vi "Facade.vi"(0 "Data In":T5, 2 "Display State In":T3, 3 "Container State":T4) -> (6 "Data Out":T5, 7 "Display State Out":T3, 8 "Action":T2)   [LabVIEW 2020, in "Advanced Stimulus Options.xctl"]
uses:
  Advanced Stimulus Options.xctl
  Advanced Stimulus Options.ctl
  <vilib>/_xctls/Container State.ctl
  State.ctl
  <vilib>/_xctls/Action.ctl
  Utility VIs/Buttons/KCheckmarkBoolean 2.ctl
  <vilib>/_xctls/XControlSupport.lvlib
panel:
  in  "Persist":T1
  in  "Alternate polarity":T1
  in  "Expression":string
  in  "Variable":u16(ring)
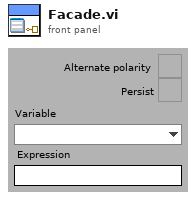
[diagram p1: front panel]
types:
  T1 = typedef "KCheckmarkBoolean 2.ctl" = bool
  T2 = typedef "XControlSupport.lvlib/Action.ctl" = cluster{"Data Changed?":bool, "State Changed?":bool, "Action Name":string}
  T3 = typedef "Advanced Stimulus Options.xctl/State.ctl" = cluster{"VarNames":string[], "show vars":bool, "show persist":bool}
  T4 = typedef "XControlSupport.lvlib/Container State.ctl" = cluster{"Indicator?":bool, "Run Mode?":bool, " Refnum":refnum<vi>}
  T5 = typedef "Advanced Stimulus Options.xctl/Advanced Stimulus Options.ctl" = cluster{"Rep Mask":string, "AltPol":bool, "Var":string, "Expr":string, "Persist":bool}
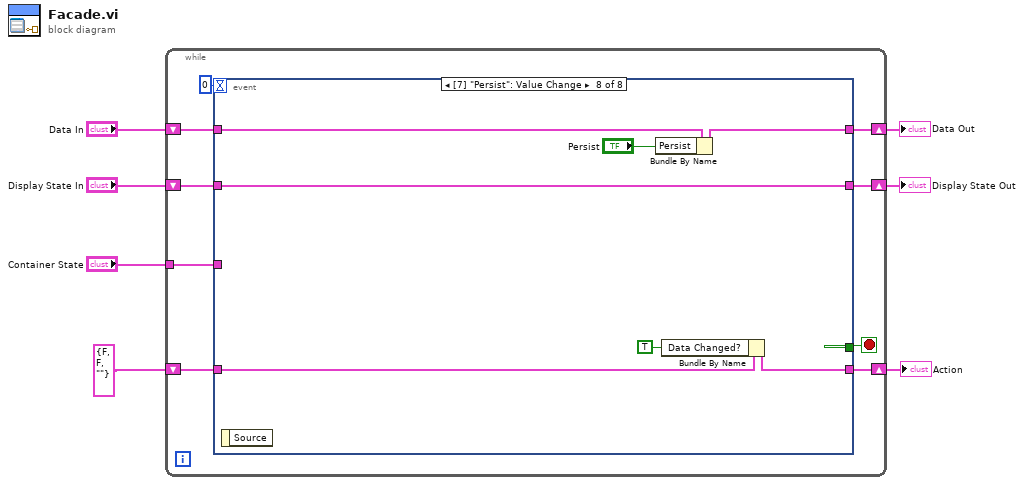
[diagram p0: block diagram]
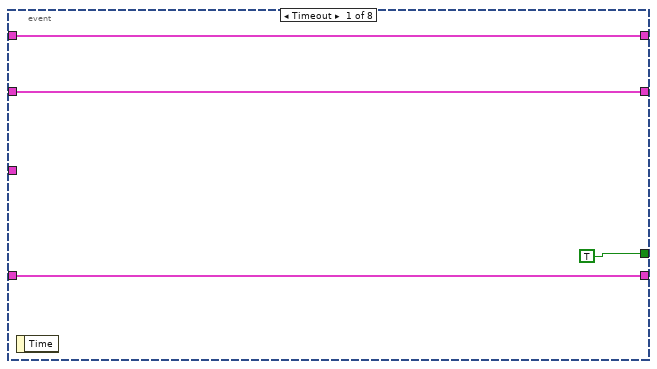
[diagram p2: hidden frame]
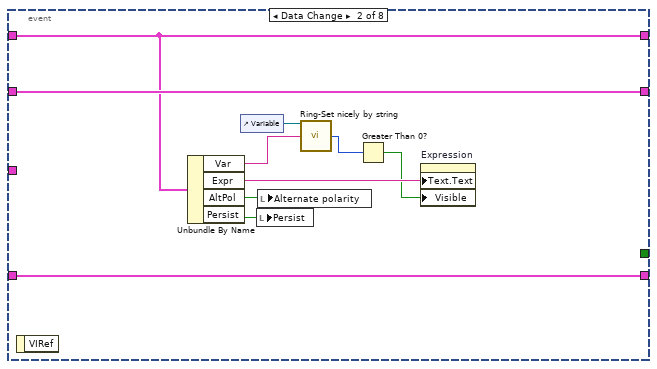
[diagram p3: hidden frame]
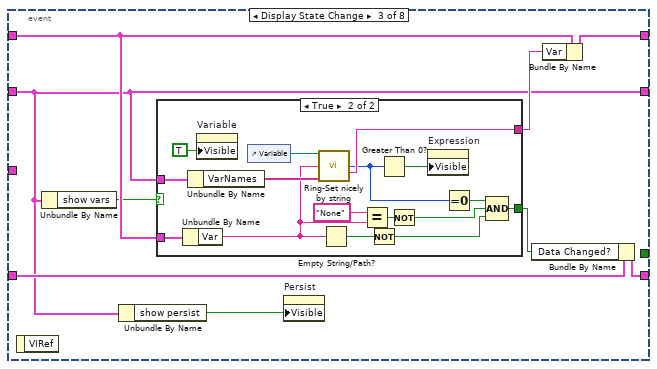
[diagram p4: hidden frame]
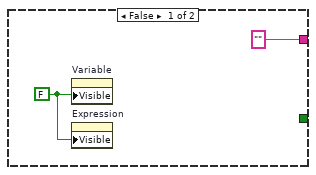
[diagram p5: hidden frame]
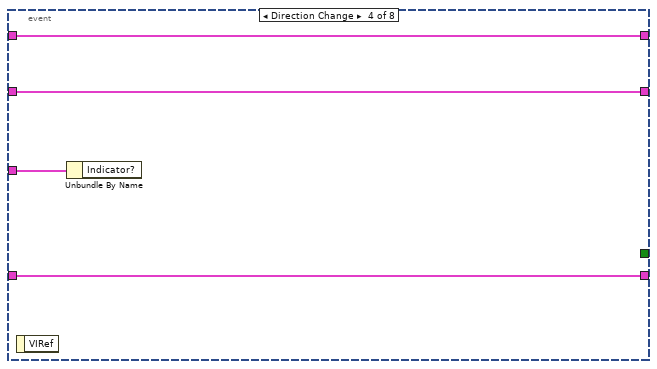
[diagram p6: hidden frame]
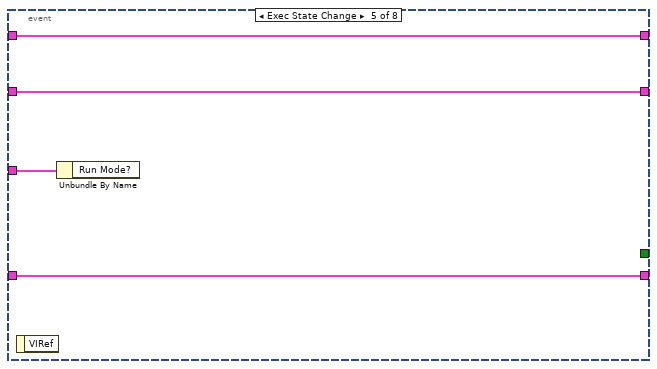
[diagram p7: hidden frame]
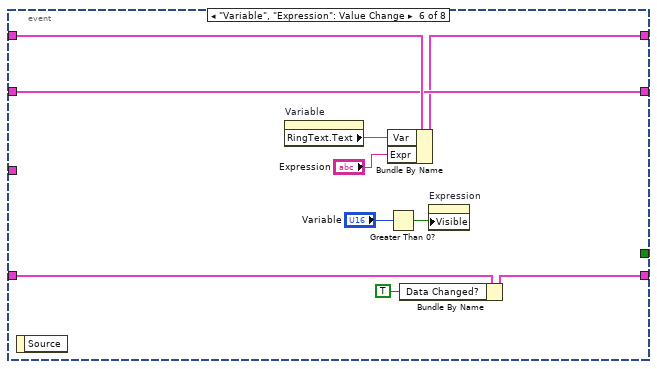
[diagram p8: hidden frame]
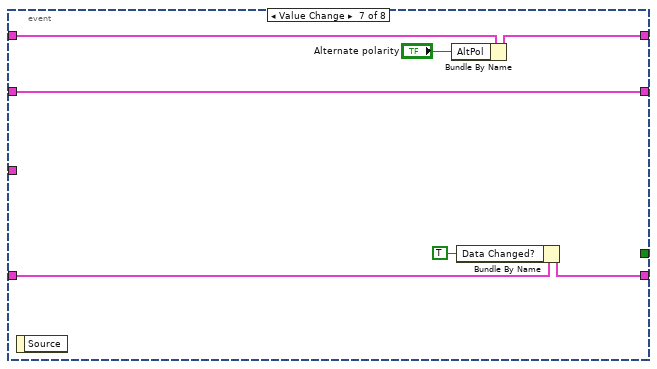
[diagram p9: hidden frame]
diagram:
  n1 = while {
    shift-right: [w15] -> w4
    shift-left: "Display State In" -> [w16]
    tunnel: "Container State" -> [w12]
    shift-right: [w10] -> w7
    shift-left: "Data In" -> [w11]
    shift-right: [w8] -> w2
    shift-left: T2 {"Data Changed?"=FALSE, "State Changed?"=FALSE, "Action Name"=""} ("Action") -> [w9]
    stop <- w14 stop-if-true
    n2 = event shown="[7] \"Persist\": Value Change" {
      selector: _ -> [_ _ _ _ _ _ _ _]
      dyn-events: _ -> [_ _ _ _ _ _ _ _]
      timeout: 0 -> [_ _ _ _ _ _ _ _]
      tunnel: w16 -> [w18 w30 w31 w60 w64 w74 w81 w88]
      tunnel: [w18 w30 w31 w60 w64 w74 w81 w88] -> w15
      tunnel: [TRUE _ _ _ _ _ _ _] -> w14
      tunnel: w12 -> [_ _ _ w61 w65 _ _ _]
      tunnel: w11 -> [w17 w27 w38 w59 w63 w75 w82 w89]
      tunnel: [w17 w27 w37 w59 w63 w72 w79 w86] -> w10
      tunnel: [w19 w29 w35 w58 w62 w71 w77 w85] -> w8
      tunnel: w9 -> [w19 w29 w39 w58 w62 w73 w80 w87]
      event Timeout {
        n3 = event-data() -> ()  [unwired: 1 in, 1 out]
      }
      event Data Change {
        n4 = event-data() -> ()  [unwired: 1 in, 1 out]
        n5 = Unbundle By Name(w27) -> ("Var"=w26:string, "Expr"=w24:string, "AltPol"=w22:bool, "Persist"=w21:bool)
        n6 = control-ref of="Variable"() -> (w28:refnum<vi>)
        n7 = local write "Persist"(w21) -> ()
        n8 = local write "Alternate polarity"(w22) -> ()
        n9 = call "Ring-Set nicely by string.vi"("Ring in"=w28, "Device"=w26) -> ("Index"=w25:i32)  [unwired: 10 in, 3 out]
        n10 = Greater Than 0?(x=w25) -> (x > 0?=w23:bool)
        n11 = property on="Expression" class="Str"("Text.Text"=w24, "Visible"=w23) -> ()  [unwired: 2 in, 2 out]
      }
      event Display State Change {
        n12 = event-data() -> ()  [unwired: 1 in, 1 out]
        n13 = Unbundle By Name(w31) -> ("show vars"=w34:bool)
        n14 = Unbundle By Name(w31) -> ("show persist"=w32:bool)
        n15 = case shown="True" w34 {
          tunnel: w31 -> [_ w57]
          tunnel: w38 -> [_ w56]
          tunnel: ["" ("Selection") w52] -> w36
          tunnel: [_ w47] -> w33
          frame False {
            w40 = FALSE
            n16 = property on="Variable" class="Ring (strict)"("Visible"=w40) -> ()  [unwired: 2 in, 2 out]
            n17 = property on="Expression" class="Str"("Visible"=w40) -> ()  [unwired: 2 in, 2 out]
          }
          frame True {
            n18 = Unbundle By Name(w56) -> ("Var"=w45:string)
            n19 = Unbundle By Name(w57) -> ("VarNames"=w54:string[])
            n20 = property on="Variable" class="Ring (strict)"("Visible"=TRUE) -> ()  [unwired: 2 in, 2 out]
            n21 = control-ref of="Variable"() -> (w55:refnum<vi>)
            n22 = call "Ring-Set nicely by string.vi"("Ring in"=w55, "Device"=w45, "Strings []"=w54) -> ("Index"=w50:i32, "Selection"=w52:string)  [unwired: 9 in, 2 out]
            n23 = Empty String/Path?(string/path=w45) -> (empty?=w48:bool)
            n24 = Equal?(x="None", y=w45) -> (x = y?=w43:bool)
            n25 = Not(x=w48) -> (.not. x?=w46:bool)
            n26 = Greater Than 0?(x=w50) -> (x > 0?=w53:bool)
            n27 = Not(x=w43) -> (.not. x?=w42:bool)
            n28 = property on="Expression" class="Str"("Visible"=w53) -> ()  [unwired: 2 in, 2 out]
            n29 = Equal To 0?(x=w50) -> (x = 0?=w49:bool)
            n30 = Compound Arithmetic op=AND(w49, w42, w46) -> (w47:bool)
          }
        }
        n31 = property on="Persist" class="Bool (strict)"("Visible"=w32) -> ()  [unwired: 2 in, 2 out]
        n32 = Bundle By Name(cluster=w39, "Data Changed?"=w33) -> (w35:T2)
        n33 = Bundle By Name(cluster=w38, "Var"=w36) -> (w37:T5)
      }
      event Direction Change {
        n34 = event-data() -> ()  [unwired: 1 in, 1 out]
        n35 = Unbundle By Name(w61) -> ()  [unwired: 1 out]
      }
      event Exec State Change {
        n36 = event-data() -> ()  [unwired: 1 in, 1 out]
        n37 = Unbundle By Name(w65) -> ()  [unwired: 1 out]
      }
      event "Variable", "Expression": Value Change {
        n38 = event-data() -> ()  [unwired: 1 in, 1 out]
        n39 = property on="Variable" class="Ring (strict)"() -> ("RingText.Text"=w69:string)  [unwired: 2 in, 2 out]
        n40 = Bundle By Name(cluster=w75, "Var"=w69, "Expr"="Expression") -> (w72:T5)
        n41 = Greater Than 0?(x="Variable") -> (x > 0?=w67:bool)
        n42 = Bundle By Name(cluster=w73, "Data Changed?"=TRUE) -> (w71:T2)
        n43 = property on="Expression" class="Str"("Visible"=w67) -> ()  [unwired: 2 in, 2 out]
      }
      event Value Change {
        n44 = event-data() -> ()  [unwired: 1 in, 1 out]
        n45 = Bundle By Name(cluster=w82, "AltPol"="Alternate polarity") -> (w79:T5)
        n46 = Bundle By Name(cluster=w80, "Data Changed?"=TRUE) -> (w77:T2)
      }
      event Value Change {
        n47 = event-data() -> ()  [unwired: 1 in, 1 out]
        n48 = Bundle By Name(cluster=w89, "Persist"="Persist") -> (w86:T5)
        n49 = Bundle By Name(cluster=w87, "Data Changed?"=TRUE) -> (w85:T2)
      }
    }
  }
  "Display State Out" <- w4
  "Data Out" <- w7
  "Action" <- w2
